vi "Main.vi"(8 "error in":errorcluster, 9 "Error Queue":refnum<queue>, 10 "Controller Queue":refnum<queue>) -> (0 "error out":errorcluster)   [LabVIEW 2020, in "Error Handler.lvlib"]
doc: "Main Vi for controller module"
uses:
  Error Handler.lvlib
  Controls/Module Message.ctl
  Controller/Controls/Application Modules.ctl
  Controller/Controls/Application Event Message.ctl
  Controller/Controls/Application Events.ctl
  Controls/Module Consummer Loop Data.ctl
  Controller/Controls/Module State.ctl
  Controls/Error Levels.ctl
  Controller/Controller.lvlib
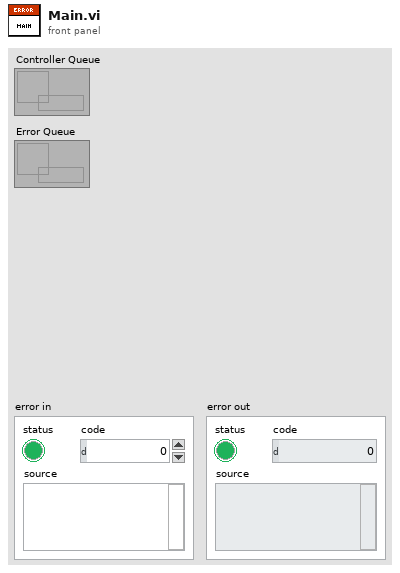
[diagram p1: front panel]
types:
  T1 = typedef "Error Handler.lvlib/Module Consummer Loop Data.ctl" = cluster{"Error File Path":path}
  T2 = typedef "Controller.lvlib/Application Event Message.ctl" = cluster{"Source":T3, "Event":T4, "Data":variant}
  T3 = typedef "Controller.lvlib/Application Modules.ctl" = enum16{"Controller", "User Console", "Display Console", "Sensor Interface", "Configuration Database", "Error Module"}
  T4 = typedef "Controller.lvlib/Application Events.ctl" = enum16{"Controller: Initialize", "Controller: Initialize Start And Move State", "Controller: Initialize Analysis State", "Controller: Initialize Continue Travel State", "Controller: Initialize Stop At Floor", "Controller: Initialize Open And Close Door Sequence", "Controller: Initialize No Request Remaining", "Controller: Initialize Emergency Call", "Controller: Initialize Terminate Process", "Controller: Publish State", "UI: Elevator Call", "UI: Broadcast State", "UI: Next Destination Reached", "UI: Timeout Reached", "UI: Emergency Call", "UI: Terminate State", "UI: Door Opened", "UI: Door Closed", "UI: Floor Reached", "UI: Door About To Close"}
  T5 = typedef "Error Handler.lvlib/Error Levels.ctl" = enum16{"Process Step", "Console Error", "Sensor Interface Error"}
  T6 = typedef "Controller.lvlib/Module State.ctl" = enum16{"Initial State", "Start And Move State", "Analysis State", "Continue Travel State", "Stop At Floor", "Open And Close Door Sequence State", "No Request Remaining State", "Emergency Call State", "Terminate Process State"}
  T7 = typedef "Error Handler.lvlib/Module Message.ctl" = cluster{"Source":T3, "Error":errorcluster}
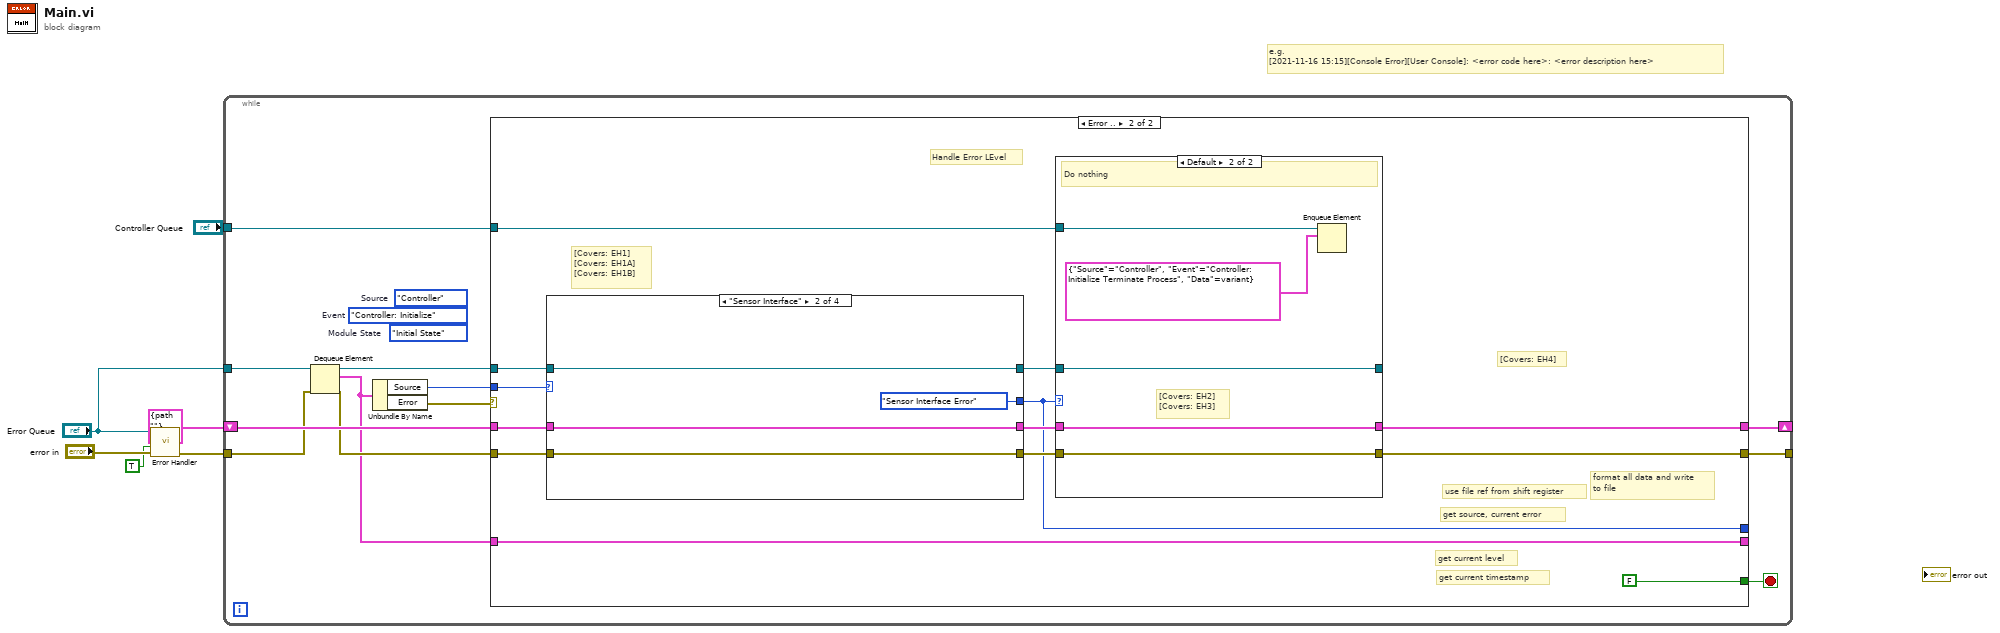
[diagram p0: block diagram]
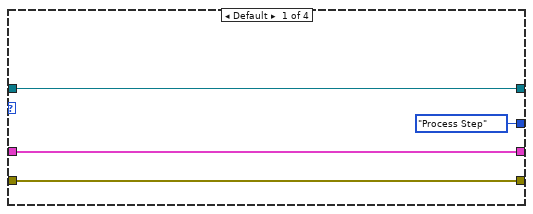
[diagram p4: hidden frame]
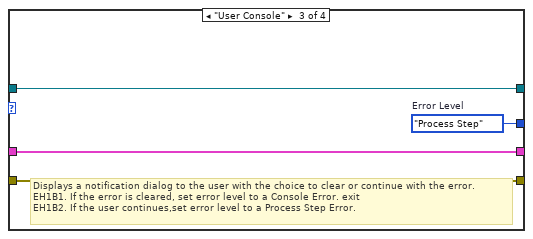
[diagram p5: hidden frame]
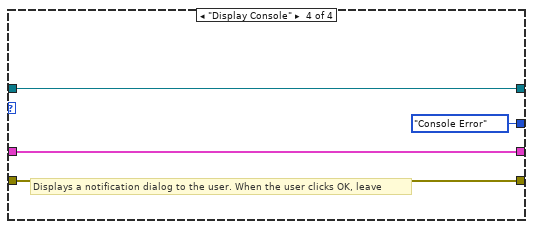
[diagram p6: hidden frame]
diagram:
  # "e.g.\n[2021-11-16 15:15][Console Error][User Console]: <error code here>: <error description here>"
  n1 = call "Error Handler.vi"("error in"="error in", "Load Reference?"=TRUE, "Error Queue"="Error Queue") -> ("error out"=w4:errorcluster)  [unwired: 8 in]
  n2 = while {
    tunnel: w4 -> [w11]
    shift-right: [w18] -> _
    shift-left: T1 {"Error File Path"=path ""} ("Loop Data") -> [w17]
    tunnel: "Error Queue" -> [w13]
    tunnel: "Controller Queue" -> [w16]
    tunnel: [w15] -> _
    stop <- w14 stop-if-true
    (unwired) Module_State."Initial State"  # Module State
    (unwired) Application_Events."Controller: Initialize"  # Event
    (unwired) Application_Modules."Controller"  # Source
    n3 = Dequeue Element(queue=w13, error in (no error)=w11) -> (queue out=w12:refnum<queue>, element=w7:T7, error out=w10:errorcluster)  [unwired: 1 in, 1 out]
    n4 = Unbundle By Name(w7) -> ("Source"=w8:T3, "Error"=w9:errorcluster)
    n5 = case shown="Error .." w9 {
      tunnel: w17 -> [w20 w29]
      tunnel: [w20 w27] -> w18
      tunnel: w12 -> [_ w32]
      tunnel: w16 -> [_ w25]
      tunnel: w10 -> [w19 w31]
      tunnel: [w19 w26] -> w15
      tunnel: [_ FALSE] -> w14
      tunnel: w8 -> [_ w23]
      tunnel: w7 -> [_ w22]
      tunnel: [_ w22] -> _
      tunnel: [_ w21] -> _
      frame #0 {
        # "Initialize error module\ncreate error file\nstore reference in shift register"
      }
      frame #1 {
        # "[Covers: EH4]"
        # "get current timestamp"
        # "format all data and write\nto file"
        # "get current level"
        # "get source, current error"
        # "use file ref from shift register"
        # "[Covers: EH1] \n[Covers: EH1A] \n[Covers: EH1B]"
        # "Handle Error LEvel"
        n6 = case shown="\"Sensor Interface\"" w23 {
          tunnel: w29 -> [w43 w47 w52 w56]
          tunnel: [w43 w47 w52 w56] -> _
          tunnel: w32 -> [w42 w46 w50 w54]
          tunnel: w31 -> [w44 w48 w51 w55]
          tunnel: [w44 w48 w51 w55] -> w28
          tunnel: [w42 w46 w50 w54] -> w30
          tunnel: [Error_Levels."Process Step" ("Error Level") Error_Levels."Sensor Interface Error" ("Error Level") w49 Error_Levels."Console Error" ("Error Level")] -> w21
          frame Default {
          }
          frame "Sensor Interface" {
          }
          frame "User Console" {
            w49 = Error_Levels."Process Step"  # Error Level
            # "Displays a notification dialog to the user with the choice to clear or continue with the error.\nEH1B1. If the error is cleared, set error level to a Console Error. exit\nEH1B2. If the user continues,set error level to a Process Step Error."
          }
          frame "Display Console" {
            # "Displays a notification dialog to the user. When the user clicks OK, leave"
          }
        }
        n7 = case shown="Default" w21 {
          tunnel: w29 -> [w34 w39]
          tunnel: [w34 w39] -> w27
          tunnel: w30 -> [w33 w38]
          tunnel: w28 -> [w35 w40]
          tunnel: [w35 w40] -> w26
          tunnel: [w33 w38] -> _
          tunnel: w25 -> [_ w37]
          frame "Console Error" {
            # "Do nothing"
          }
          frame Default {
            # "[Covers: EH2] \n[Covers: EH3]"
            # "Do nothing"
            n8 = Enqueue Element(queue=w37, element=T2 {"Source"=enum."Controller", "Event"=enum."Controller: Initialize Terminate Process", "Data"=variant}) -> ()  [unwired: 2 in, 3 out]
          }
        }
      }
    }
  }
